vi "Status Query.vi"(0 "VISA resource name":refnum<visa-resource-name>, 11 "error in (no error)":errorcluster) -> (1 "OK or warning":bool, 3 "SRQ":bool, 4 "VISA resource name out":refnum<visa-resource-name>, 6 "Measurement message":string, 8 "Status code":u16, 10 "Status byte":bool[](array[boolean]), 12 "Error":bool, 14 "Syntax error":bool, 15 "error out":errorcluster)   [LabVIEW 2020, in "Datron D4xxx.lvlib"]
doc: "Queries the instrument status."
uses:
  Datron D4xxx.lvlib
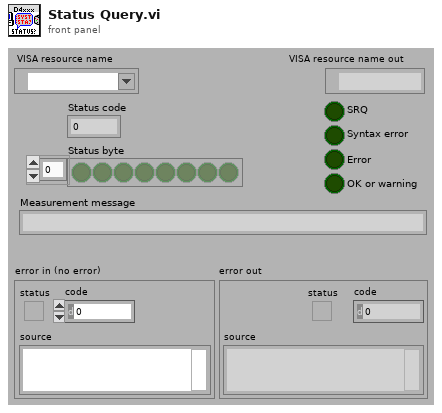
[diagram p1: front panel]
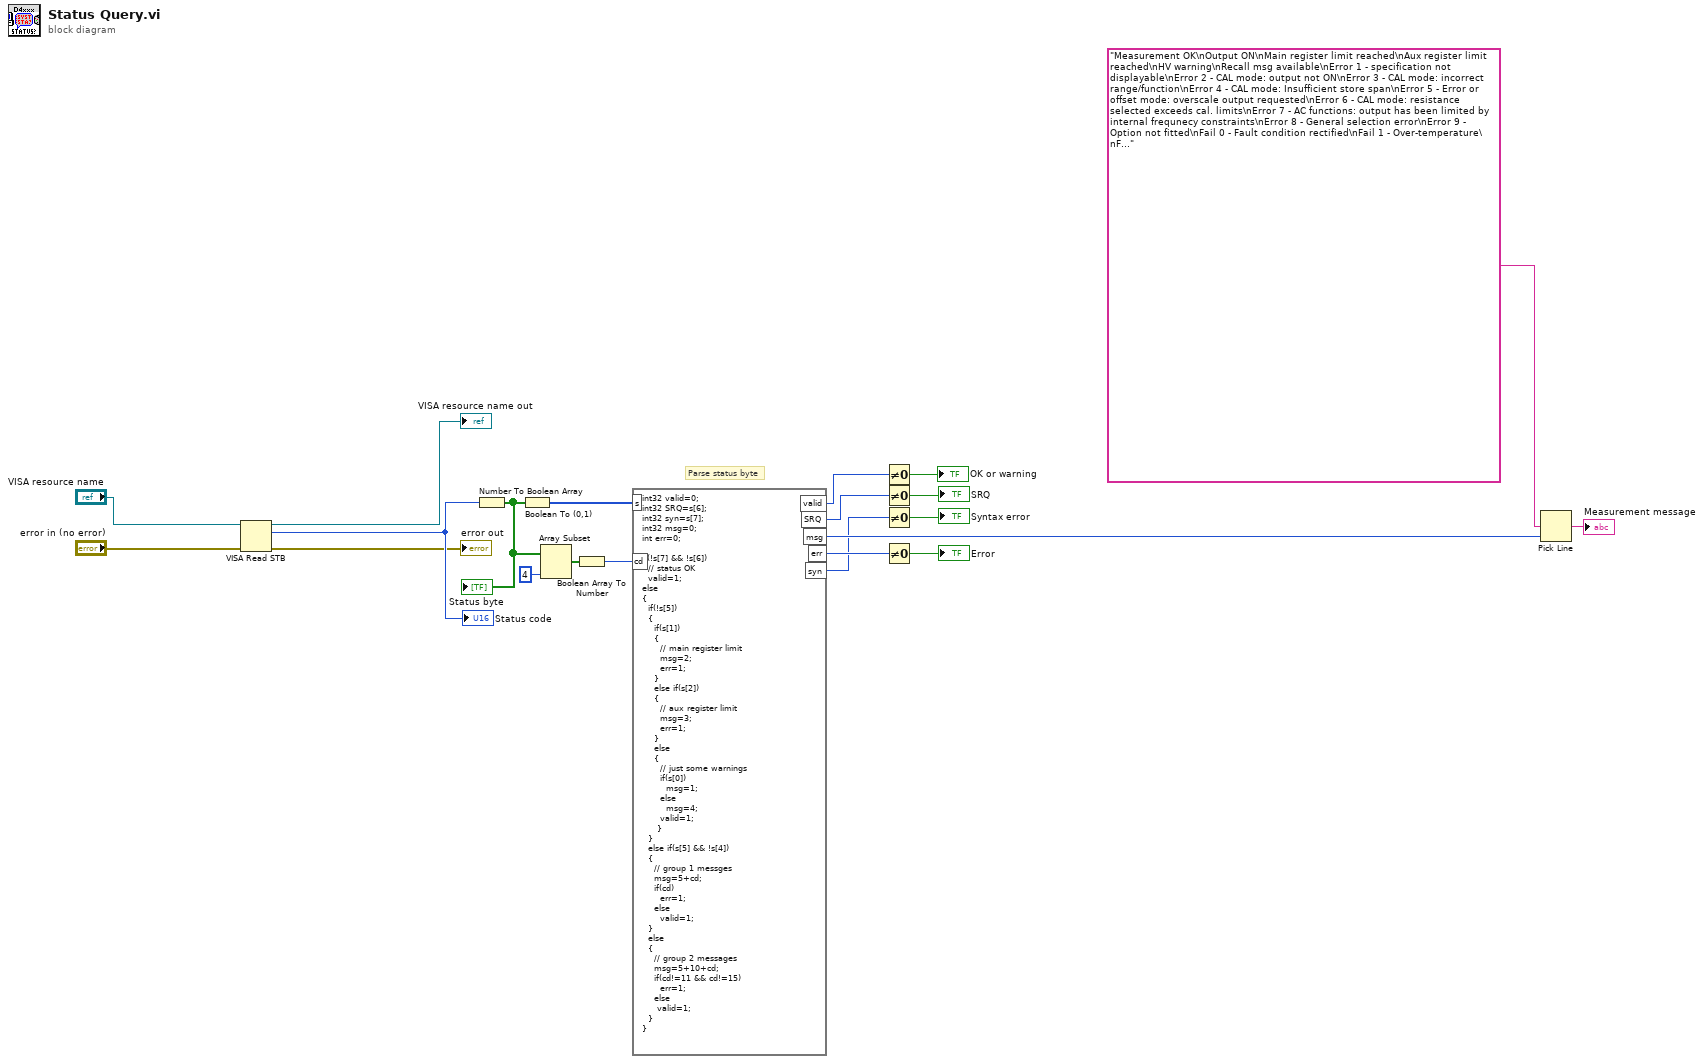
[diagram p0: block diagram]
diagram:
  # "Parse status byte"
  n1 = VISA Read STB(8:"error in (no error)", 11:"VISA resource name") -> (0:→"error out":errorcluster, 2:w20:u16, 3:→"VISA resource name out":refnum<visa-resource-name>)
  "Status code" <- w20
  n2 = Number To Boolean Array(number=w20) -> (Boolean array=w13:bool[])
  "Status byte" <- w13
  n3 = Boolean To (0,1)(Boolean=w13) -> (0, 1=w18:i16[])
  n4 = Array Subset(array=w13, length=4) -> (w11:bool[])  [unwired: 1 in]
  n5 = Boolean Array To Number(Boolean array=w11) -> (number=w10:u32)
  n6 = formula code="int32 valid=0;\nint32 SRQ=s[6];\nint32 syn=s[7];\nint32 msg=0;\nint err=0;\n\nif(!s[7] && !s[6])\n  // status OK\n  valid=1;\nelse\n{\n  if(!s[5])\n  {\n    if(s[1])\n    {\n      // main register limit\n      msg=2;\n      err=1;\n    }\n    else if(s[2])\n    {\n      // aux register limit\n      msg=3;\n      err=1;\n    }\n    else\n    {\n      // just some warnings\n      if(s[0])\n        msg=1;\n      else\n        msg=4;\n      valid=1;\n     }\n  }\n  else if(s[5] && !s[4])\n  {\n    // group 1 messges\n    msg=5+cd;\n    if(cd)\n      err=1;\n    else\n      valid=1;\n  }\n  else\n  {\n    // group 2 messages\n    msg=5+10+cd;\n    if(cd!=11 && cd!=15)\n      err=1;\n    else\n     valid=1;\n  }\n}"("s"=w18, "cd"=w10) -> ("valid"=w17:i32, "SRQ"=w14:i32, "msg"=w7:i32, "err"=w6:i32, "syn"=w3:i32)
  n7 = Not Equal To 0?(x=w17) -> (x != 0?=→"OK or warning":bool)
  n8 = Not Equal To 0?(x=w14) -> (x != 0?=→"SRQ":bool)
  n9 = Not Equal To 0?(x=w3) -> (x != 0?=→"Syntax error":bool)
  n10 = Not Equal To 0?(x=w6) -> (x != 0?=→"Error":bool)
  n11 = Pick Line(multi-line string="Measurement OK\nOutput ON\nMain register limit reached\nAux register limit reached\nHV warning\nRecall msg available\nError 1 - specification not displayable\nError 2 - CAL mode: output not ON\nError 3 - CAL mode: incorrect range/function\nError 4 - CAL mode: Insufficient store span\nError 5 - Error or offset mode: overscale output requested\nError 6 - CAL mode: resistance selected exceeds cal. limits\nError 7 - AC functions: output has been limited by internal frequnecy constraints\nError 8 - General selection error\nError 9 - Option not fitted\nFail 0 - Fault condition rectified\nFail 1 - Over-temperature\nFail 2 - Over-voltage\nFail 3 - Control data currupted\nFail 4 - Precision divider fault\nFail 5 - Safety alarm\nFail 6 - Cal. store sum check non-parity\nFail 7 - 400V power supply fault\nFail 8 - 38V power supply fault\nFail 9 - 15V in-guard power supply fault\nFail 10 - Model 4600 communication fault or option 70 fault\nRest. Instrument reset to power-up state\nError EF. External frequency not present\nSpot frequency not calibrated\nOverload - Current or voltage limit\nPower-on", line index=w7) -> (output string=→"Measurement message":string)  [unwired: 1 in]
